vi "arrayConvert.vi"(0 "输入数组":dbl[](array[numeric])) -> (1 "ch0":dbl[](array[numeric]), 2 "ch1":dbl[](array[numeric]))   [LabVIEW 2018]
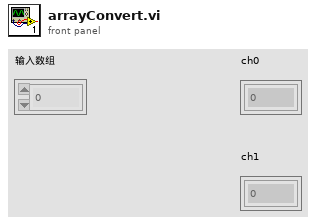
[diagram p1: front panel]
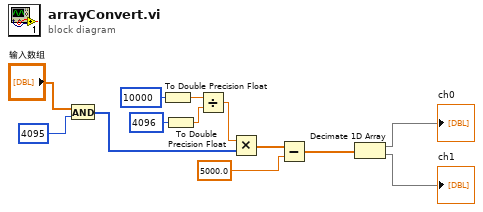
[diagram p0: block diagram]
diagram:
  n1 = And(x="输入数组", y=u16 4095) -> (x .and. y?=w5:i32[])
  n2 = To Double Precision Float(number=10000 ("x")) -> (double precision float=w12:dbl)
  n3 = To Double Precision Float(number=4096) -> (double precision float=w11:dbl)
  n4 = Divide(x=w12, y=w11) -> (x/y=w9:dbl)
  n5 = Multiply(x=w9, y=w5) -> (x*y=w10:dbl[])
  n6 = Subtract(x=w10, y=5000.0) -> (x-y=w3:dbl[])
  n7 = Decimate 1D Array(w3) -> (→"ch0":dbl[], →"ch1":dbl[])
